vi "To String.vi"(11 "JSON Array in":refnum<class "JSON Array.lvclass">) -> (2 "String":string)   [LabVIEW 2017, in "LVJSON.lvlib" / "JSON Array.lvclass"]
uses:
  JSON Array.lvclass
  JSON Array.lvclass/JSON Array.ctl
  JSON Datatype/JSON Datatype.lvclass
  LVJSON.lvlib
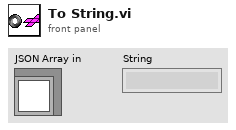
[diagram p1: front panel]
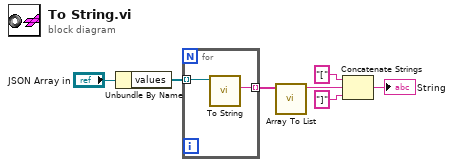
[diagram p0: block diagram]
diagram:
  n1 = Unbundle By Name("JSON Array in") -> ("values"=w6:refnum<class "JSON Datatype.lvclass">[])
  n2 = for {
    tunnel: w6 -> [w9] mode=indexing
    tunnel: [w8] -> w2 mode=indexing
    n3 = call-dynamic "To String.vi"("JSON Datatype in"=w9) -> ("String"=w8:string)  [unwired: 10 in]
  }
  n4 = call "Array To List.vi"("Array"=w2) -> ("String"=w1:string)  [unwired: 10 in]
  n5 = Concatenate Strings("[" ("string"), w1, "]" ("string")) -> (→"String":string)
